vi "correccionrotacion.vi"(2 "Patron original":T1, 3 "Toma original":T1) -> (0 "Patron original (dupl)":T1(plugin-control) caption="Perfil lateral", 1 "Toma rotada":T1(plugin-control) caption="Perfil lateral")   [LabVIEW 2021]
doc: "Rota una imagen con respeco a otra a partir de sus centroides"
uses:
  <vilib>/vision/Image Controls.llb/IMAQ Image.ctl
  <vilib>/vision/NI_Vision_Development_Module.lvlib
panel:
  out "Angle (deg)":dbl format="%.2f"
  out "Toma original":T1(plugin-control) caption="Perfil lateral"
  # "CUEVAS CERÓN SERGIO ALBERTO\nREYES PÉREZ JAVIER\nSALCEDO LICEA JUAN CARLOS"
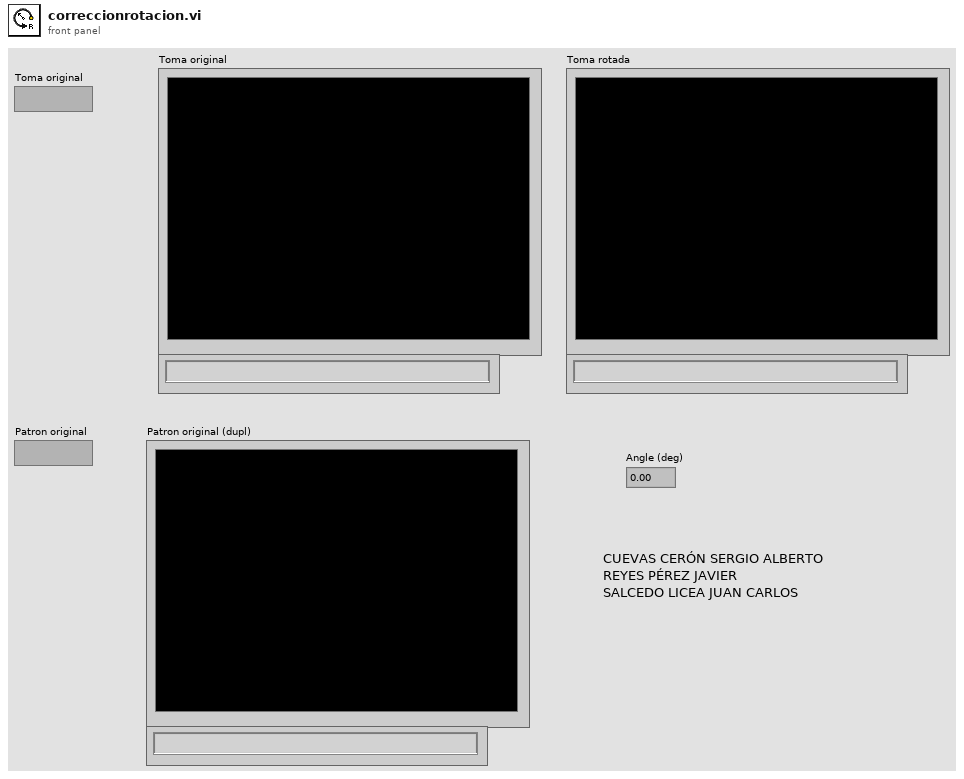
[diagram p1: front panel]
types:
  T1 = typedef "IMAQ Image.ctl" = refnum<image>
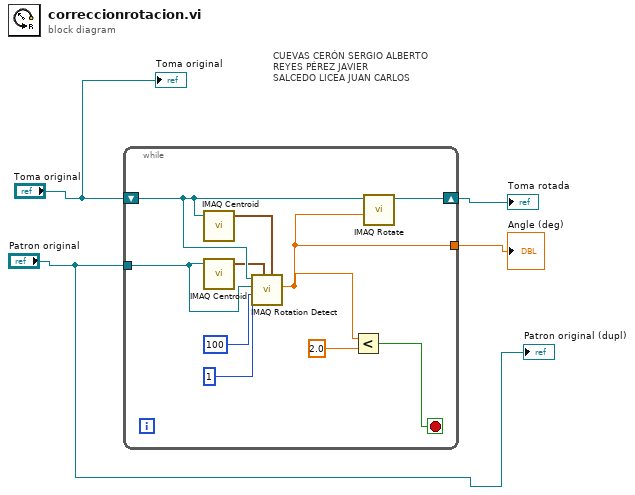
[diagram p0: block diagram]
diagram:
  # "CUEVAS CERÓN SERGIO ALBERTO\nREYES PÉREZ JAVIER\nSALCEDO LICEA JUAN CARLOS"
  n1 = while {
    tunnel: "Patron original" -> [w10]
    shift-right: [w12] -> w3
    shift-left: "Toma original" -> [w11]
    tunnel: [w5] -> w1
    stop <- w8 stop-if-true
    n2 = call "IMAQ Centroid"("Image"=w11) -> ("Centroid"=w7:cluster{"X Centroid":sgl, "Y Centroid":sgl})  [unwired: 3 in, 1 out]
    n3 = call "IMAQ Centroid"("Image"=w10) -> ("Centroid"=w6:cluster{"X Centroid":sgl, "Y Centroid":sgl})  [unwired: 3 in, 1 out]
    n4 = call "IMAQ Rotation Detect"("Reference Center"=w7, "Precision (degrees)"=1, "Image 2 Center"=w6, "Radius"=100, "Image 2"=w10, "Reference Image"=w11) -> ("Angle (deg)"=w5:dbl)  [unwired: 3 in, 2 out]
    n5 = Less?(x=w5, y=2.0) -> (x < y?=w8:bool)
    n6 = call "IMAQ Rotate"("Angle (degrees)"=w5, "Image Src"=w11) -> ("Image Dst Out"=w12:T1)  [unwired: 8 in, 1 out]
  }
  "Toma rotada" <- w3
  "Angle (deg)" <- w1
  "Patron original (dupl)" <- "Patron original"
  "Toma original" <- "Toma original"
